vi "Command2Cluster.vi"(8 "error in":errorcluster, 11 "Current command":string) -> (0 "error out":errorcluster, 3 "Cluster":T1 {"Green-Red" step=1 scale=0.0..100.0; "Blue" step=1 scale=0.0..100.0; "Violet" step=1 scale=0.0..100.0})   [LabVIEW 2025]
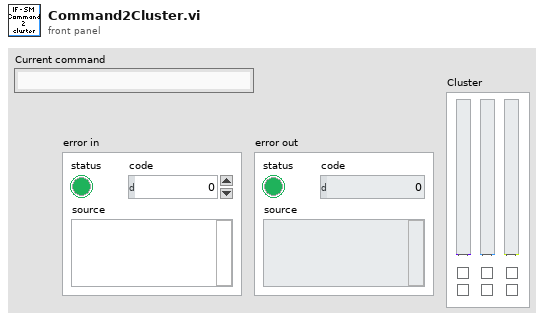
[diagram p1: front panel]
types:
  T1 = cluster{"Violet":u8, "Blue":u8, "Green-Red":u8, "A(S)Selected/(N)Unselected":bool, "B(S)Selected/(N)Unselected":bool, "C(S)Selected/(N)Unselected":bool, "A(N)ON/(F)OFF":bool, "(N)ON/(F)OFF":bool, "C(N)ON/(F)OFF":bool}
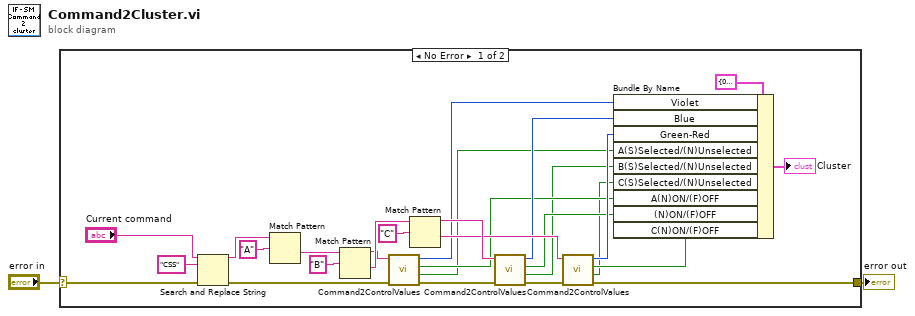
[diagram p0: block diagram]
diagram:
  n1 = case shown="No Error" "error in" {
    selector: "error in" -> [w28 w30]
    tunnel: [w16 w30] -> w1
    frame No Error {
      n2 = Search and Replace String(input string="Current command", search string="CSS", error in=w28) -> (result string=w26:string, error out=w19:errorcluster)  [unwired: 5 in, 2 out]
      n3 = Match Pattern(string=w26, regular expression="A") -> (after substring=w23:string)  [unwired: 1 in, 3 out]
      n4 = Match Pattern(string=w23, regular expression="B") -> (before substring=w20:string, after substring=w21:string)  [unwired: 1 in, 2 out]
      n5 = call "Command2ControlValues.vi"("error in"=w19, "Command"=w20) -> ("error out"=w18:errorcluster, "(S)Selected/(N)Unselected"=w5:bool, "(N)ON/(F)OFF"=w8:bool, "Intensity"=w11:u8)  [unwired: 6 in]
      n6 = Match Pattern(string=w21, regular expression="C") -> (before substring=w15:string, after substring=w14:string)  [unwired: 1 in, 2 out]
      n7 = call "Command2ControlValues.vi"("error in"=w18, "Command"=w15) -> ("error out"=w17:errorcluster, "(S)Selected/(N)Unselected"=w4:bool, "(N)ON/(F)OFF"=w7:bool, "Intensity"=w10:u8)  [unwired: 6 in]
      n8 = call "Command2ControlValues.vi"("error in"=w17, "Command"=w14) -> ("error out"=w16:errorcluster, "(S)Selected/(N)Unselected"=w3:bool, "(N)ON/(F)OFF"=w6:bool, "Intensity"=w9:u8)  [unwired: 6 in]
      n9 = Bundle By Name(cluster=T1 {"Violet"=0, "Blue"=0, "Green-Red"=0, "A(S)Selected/(N)Unselected"=FALSE, "B(S)Selected/(N)Unselected"=FALSE, "C(S)Selected/(N)Unselected"=FALSE, "A(N)ON/(F)OFF"=FALSE, "(N)ON/(F)OFF"=FALSE, "C(N)ON/(F)OFF"=FALSE} ("Cluster"), "Violet"=w11, "Blue"=w10, "Green-Red"=w9, "A(S)Selected/(N)Unselected"=w5, "B(S)Selected/(N)Unselected"=w4, "C(S)Selected/(N)Unselected"=w3, "A(N)ON/(F)OFF"=w8, "(N)ON/(F)OFF"=w7, "C(N)ON/(F)OFF"=w6) -> (→"Cluster":T1)
    }
    frame Error {
    }
  }
  "error out" <- w1
